vi "CalculateTriggerState.vi"(10 "Previous Trigger Value":dbl, 11 "Current Trigger Value":dbl) -> (1 "End Triggered/Close?":bool, 2 "Triggered/Logging?":bool, 3 "Just Triggered/Setup?":bool)   [LabVIEW 2024, in "Embedded TDMS Logger Engine.lvlib" / "Channel Manager.lvclass"]
doc: "Determines whether the trigger state has just changed, whether it be on the rising or falling edge to determine:\n- Have we just triggered?\n- Have we gone from triggered to not in the last iteration?\n- Are we currently triggered?\n\nThis is useful for knowing whether to immediately open a new file, close the current, log or do nothing."
uses:
  Channel Reader/Channel Manager.lvclass
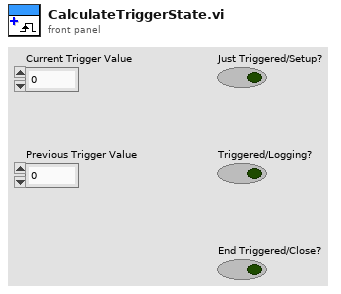
[diagram p1: front panel]
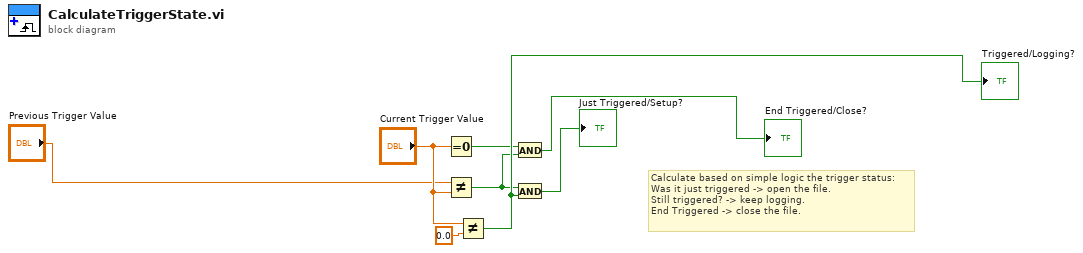
[diagram p0: block diagram]
diagram:
  # "Calculate based on simple logic the trigger status:\nWas it just triggered -> open the file.\nStill triggered? -> keep logging.\nEnd Triggered -> close the file."
  n1 = Equal To 0?(x="Current Trigger Value") -> (x = 0?=w4:bool)
  n2 = Not Equal?(x="Previous Trigger Value", y="Current Trigger Value") -> (x != y?=w5:bool)
  n3 = Not Equal?(x="Current Trigger Value", y=0.0) -> (x != y?=w7:bool)
  "Triggered/Logging?" <- w7
  n4 = And(x=w4, y=w5) -> (x .and. y?=→"End Triggered/Close?":bool)
  n5 = And(x=w5, y=w7) -> (x .and. y?=→"Just Triggered/Setup?":bool)
